vi "main.vi"() -> ()   [LabVIEW 2017]
uses:
  <vilib>/Instr/_visa.llb/VISA Configure Serial Port (Instr).vi
  <vilib>/Utility/file.llb/Write Delimited Spreadsheet (DBL).vi
  <vilib>/ptbypt/NI_PtbyPt.lvlib
panel:
  out "路径":path
  out "XY图":cluster{dbl[], dbl[]}(graph)
  out "激光位移传感器":dbl(graph)
  in  "模拟信号串口号":refnum<visa-resource-name>="COM12"
  out "读取缓冲区 2":string
  out "力传感器":cluster{dbl, dbl, dbl}(graph)
  out "Fz":dbl
  out "Fy":dbl
  out "Fx":dbl
  out "连接的字符串":string
  out "频率/Hz":dbl
  out "relative seconds":dbl caption="相对秒钟" format="%_19f"
  in  "六轴力传感器置零":bool
  in  "停止":bool
  in  "六轴力传感器串口号":refnum<visa-resource-name>="COM11"
  out "读取缓冲区":string
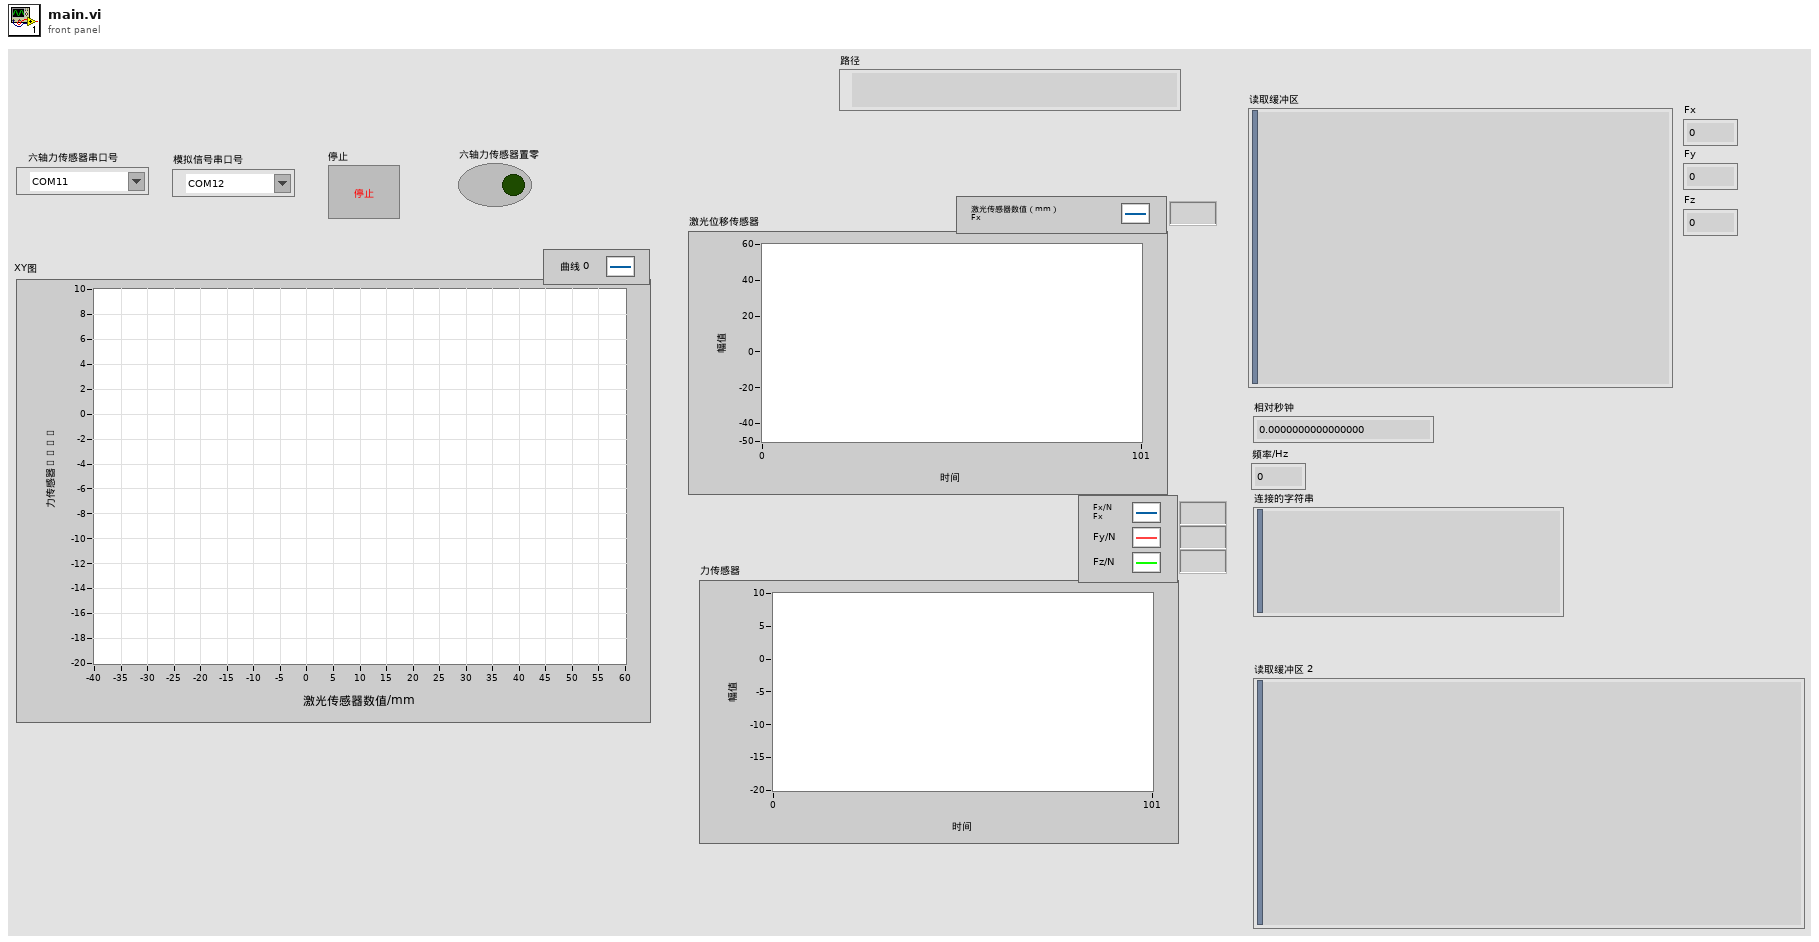
[diagram p1: front panel]
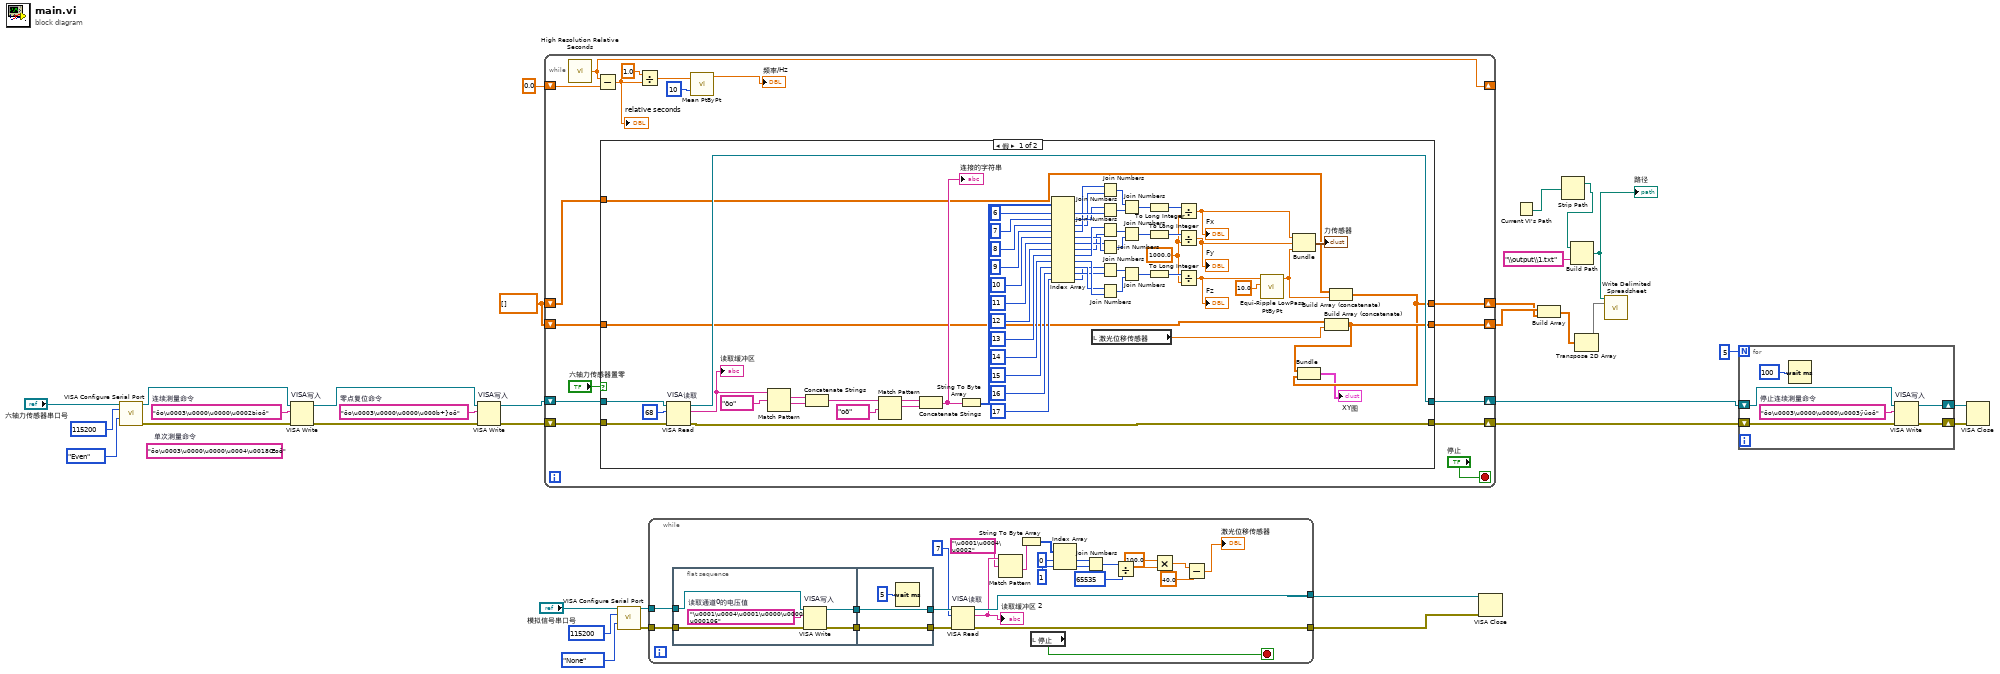
[diagram p0: block diagram]
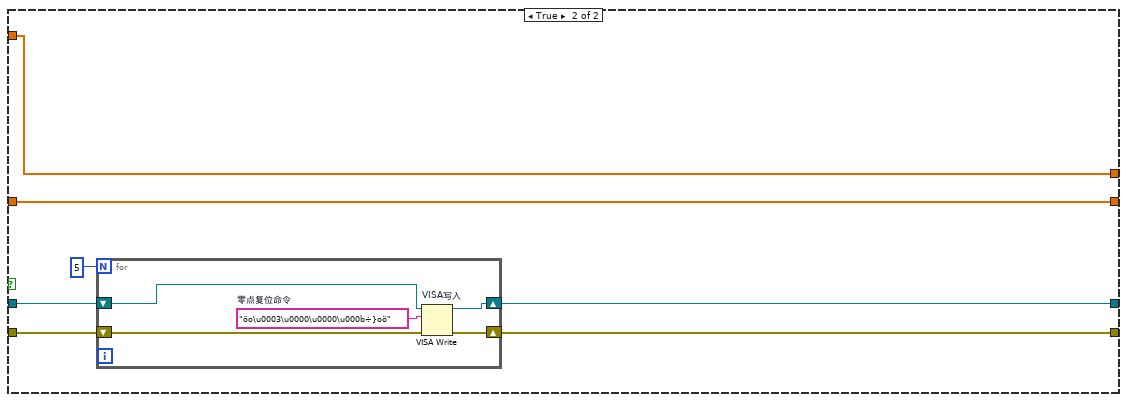
[diagram p2: hidden frame]
diagram:
  w9 = dbl[] []
  (unwired) "öo\u0003\u0000\u0000\u0004\u0018Œoö"  # 单次测量命令
  w23 = "öo\u0003\u0000\u0000\u000b÷}oö"  # 零点复位命令
  w17 = "öo\u0003\u0000\u0000\u0002Þìoö"  # 连续测量命令
  n1 = call-poly "VISA Configure Serial Port"("VISA resource name"="六轴力传感器串口号", "baud rate (9600)"=u32 115200, "parity (0:none)"=enum16{"None", "Odd", "Even", "Mark", "Space"}."Even") -> ("VISA resource name out"=w19:refnum<visa-resource-name>, "error out"=w21:errorcluster)  [unwired: 11 in]
  n2 = VISA Write "VISA写入"(VISA resource name=w19, write buffer=w17, error in (no error)=w21) -> (VISA resource name out=w18:refnum<visa-resource-name>, error out=w20:errorcluster)  [unwired: 1 out]
  n3 = VISA Write "VISA写入"(VISA resource name=w18, write buffer=w23, error in (no error)=w20) -> (VISA resource name out=w25:refnum<visa-resource-name>, error out=w24:errorcluster)  [unwired: 1 out]
  n4 = while {
    shift-right: [w50] -> w30
    shift-left: w25 -> [w39]
    shift-right: [w49] -> w29
    shift-left: w24 -> [w38]
    shift-right: [w46] -> _
    shift-left: 0.0 ("relative seconds") -> [w45]
    shift-right: [w37] -> w7
    shift-left: w9 -> [w36]
    shift-right: [w35] -> w8
    shift-left: w9 -> [w34]
    stop <- "停止" stop-if-true
    n5 = call <vilib>:"High Resolution Relative Seconds.vi"() -> ("relative seconds"=w46:dbl)
    n6 = Subtract(x=w46, y=w45) -> (x-y=w44:dbl)
    "relative seconds" <- w44
    n7 = case shown="假" "六轴力传感器置零" {
      tunnel: [w113 w120] -> w50
      tunnel: [w112 w121] -> w49
      tunnel: w39 -> [w59 w118]
      tunnel: w38 -> [w58 w117]
      tunnel: [w52 w116] -> w37
      tunnel: w36 -> [w56 w116]
      tunnel: [w53 w115] -> w35
      tunnel: w34 -> [w54 w115]
      frame False {
        w76 = 1000.0
        n8 = VISA Read "VISA读取"(VISA resource name=w59, byte count=u32 68 ("字节总数"), error in (no error)=w58) -> (VISA resource name out=w113:refnum<visa-resource-name>, read buffer=w111:string, error out=w112:errorcluster)  [unwired: 1 out]
        "读取缓冲区" <- w111
        n9 = Match Pattern(string=w111, regular expression="öo" ("正则表达式")) -> (match substring=w107:string, after substring=w106:string)  [unwired: 1 in, 2 out]
        n10 = Concatenate Strings(w107, w106) -> (w105:string)
        n11 = Match Pattern(string=w105, regular expression="oö" ("正则表达式")) -> (before substring=w103:string, match substring=w102:string)  [unwired: 1 in, 2 out]
        n12 = Concatenate Strings(w103, w102) -> (w101:string)
        "连接的字符串" <- w101
        n13 = String To Byte Array(string=w101) -> (unsigned byte array=w109:u8[])
        n14 = Index Array(array=w109, index #1=6 ("索引"), index #2=7 ("索引"), index #3=8 ("索引"), index #4=9 ("索引"), index #5=10 ("索引"), index #6=11 ("索引"), index #7=12 ("索引"), index #8=13 ("索引"), index #9=14 ("索引"), index #10=15 ("索引"), index #11=16 ("索引"), index #12=17 ("索引")) -> (element #1=w100:u8, element #2=w99:u8, element #3=w97:u8, element #4=w98:u8, element #5=w90:u8, element #6=w89:u8, element #7=w88:u8, element #8=w91:u8, element #9=w83:u8, element #10=w82:u8, element #11=w81:u8, element #12=w80:u8)
        n15 = local read "激光位移传感器"() -> (w55:dbl)
        n16 = Join Numbers(hi=w98, lo=w97) -> ((hi.lo)=w95:u16)
        n17 = Join Numbers(hi=w99, lo=w100) -> ((hi.lo)=w96:u16)
        n18 = Join Numbers(hi=w91, lo=w88) -> ((hi.lo)=w93:u16)
        n19 = Join Numbers(hi=w89, lo=w90) -> ((hi.lo)=w92:u16)
        n20 = Join Numbers(hi=w80, lo=w81) -> ((hi.lo)=w84:u16)
        n21 = Join Numbers(hi=w82, lo=w83) -> ((hi.lo)=w85:u16)
        n22 = Join Numbers(hi=w95, lo=w96) -> ((hi.lo)=w94:u32)
        n23 = Join Numbers(hi=w93, lo=w92) -> ((hi.lo)=w87:u32)
        n24 = Join Numbers(hi=w84, lo=w85) -> ((hi.lo)=w86:u32)
        n25 = To Long Integer(number=w94) -> (32bit integer=w79:i32)
        n26 = To Long Integer(number=w87) -> (32bit integer=w77:i32)
        n27 = To Long Integer(number=w86) -> (32bit integer=w78:i32)
        n28 = Divide(x=w79, y=w76) -> (x/y=w63:dbl)
        "Fx" <- w63
        n29 = Divide(x=w77, y=w76) -> (x/y=w62:dbl)
        "Fy" <- w62
        n30 = Divide(x=w78, y=w76) -> (x/y=w61:dbl)
        "Fz" <- w61
        n31 = call <vilib>:"Equi-Ripple LowPass PtByPt.vi"("sampling freq: fs"=10.0, "x"=w61) -> ("Filtered x"=w57:dbl)  [unwired: 7 in, 1 out]
        n32 = Bundle(w63, w62, "Filtered x"=w57) -> (→"力传感器":cluster{dbl, dbl, "Filtered x":dbl})  [unwired: 1 in]
        n33 = Build Array (concatenate)(w54, w55) -> (w53:dbl[])
        n34 = Build Array (concatenate)(w56, w57) -> (w52:dbl[])
        n35 = Bundle(w53, w52) -> (→"XY图":cluster{dbl[], dbl[]})  [unwired: 1 in]
      }
      frame True {
        n36 = for {
          N: 5 -> [_]
          shift-right: [w124] -> w121
          shift-left: w117 -> [w125]
          shift-right: [w122] -> w120
          shift-left: w118 -> [w123]
          w126 = "öo\u0003\u0000\u0000\u000b÷}oö"  # 零点复位命令
          n37 = VISA Write "VISA写入"(VISA resource name=w123, write buffer=w126, error in (no error)=w125) -> (VISA resource name out=w122:refnum<visa-resource-name>, error out=w124:errorcluster)  [unwired: 1 out]
        }
      }
    }
    n38 = Divide(x=1.0, y=w44) -> (x/y=w42:dbl)
    n39 = call <vilib>:"Mean PtByPt.vi"("x"=w42, "sample length"=10) -> ("mean"=→"频率/Hz":dbl)  [unwired: 2 in, 1 out]
  }
  n40 = call-poly "VISA Configure Serial Port"("VISA resource name"="模拟信号串口号", "baud rate (9600)"=u32 115200, "parity (0:none)"=enum16{"None", "Odd", "Even", "Mark", "Space"}."None") -> ("VISA resource name out"=w13:refnum<visa-resource-name>, "error out"=w12:errorcluster)  [unwired: 11 in]
  n41 = while {
    tunnel: w13 -> [w148]
    tunnel: w12 -> [w147]
    tunnel: [w146] -> w11
    tunnel: [w145] -> w10
    stop <- w142 stop-if-true
    n42 = flat-sequence {
      tunnel: w148 -> [w153]
      tunnel: w147 -> [w152]
      tunnel: [w156] -> w144
      tunnel: [w155] -> w143
      tunnel: w144 -> [w159]
      tunnel: w143 -> [w158]
      tunnel: [w159] -> w151
      tunnel: [w158] -> w150
      frame #0 {
        w154 = "\u0001\u0004\u0001\u0000\u0000\u000106"  # 读取通道0的电压值
        n43 = VISA Write "VISA写入"(VISA resource name=w153, write buffer=w154, error in (no error)=w152) -> (VISA resource name out=w155:refnum<visa-resource-name>, error out=w156:errorcluster)  [unwired: 1 out]
      }
      frame #1 {
        n44 = Wait (ms)(milliseconds to wait=u32 5 ("等待时间（毫秒）")) -> ()  [unwired: 1 out]
      }
    }
    n45 = VISA Read "VISA读取"(VISA resource name=w150, byte count=u32 7 ("字节总数"), error in (no error)=w151) -> (VISA resource name out=w146:refnum<visa-resource-name>, read buffer=w141:string, error out=w145:errorcluster)  [unwired: 1 out]
    "读取缓冲区 2" <- w141
    n46 = Match Pattern(string=w141, regular expression="\u0001\u0004\u0002" ("正则表达式")) -> (after substring=w137:string)  [unwired: 1 in, 3 out]
    n47 = String To Byte Array(string=w137) -> (unsigned byte array=w136:u8[])
    n48 = local read "停止"() -> (w142:bool)
    n49 = Index Array(array=w136, index #1=0 ("索引"), index #2=1 ("索引")) -> (element #1=w134:u8, element #2=w135:u8)
    n50 = Join Numbers(hi=w134, lo=w135) -> ((hi.lo)=w133:u16)
    n51 = Divide(x=w133, y=u16 65535) -> (x/y=w131:dbl)
    n52 = Multiply(x=100.0, y=w131) -> (x*y=w129:dbl)
    n53 = Subtract(x=w129, y=40.0) -> (x-y=→"激光位移传感器":dbl)
  }
  n54 = VISA Close(VISA resource name=w11, error in (no error)=w10) -> ()  [unwired: 1 out]
  n55 = Current VI's Path() -> (path=w3:path)
  n56 = Build Array(w8, w7) -> (w6:dbl[][])
  n57 = Strip Path(path=w3) -> (stripped path=w2:path)  [unwired: 1 out]
  n58 = Build Path(base path=w2, name or relative path="\\output\\1.txt" ("名称或相对路径")) -> (appended path=w1:path)
  "路径" <- w1
  n59 = Transpose 2D Array(2D array=w6) -> (transposed array=w5:dbl[][])
  n60 = call-poly <vilib>:"Write Delimited Spreadsheet.vi"("file path (dialog if empty)"=w1, "2D data"=w5) -> ()  [unwired: 12 in, 2 out]
  n61 = for {
    N: 5 -> [_]
    shift-right: [w162] -> w27
    shift-left: w30 -> [w165]
    shift-right: [w163] -> w28
    shift-left: w29 -> [w164]
    w161 = "öo\u0003\u0000\u0000\u0003ÿüoö"  # 停止连续测量命令
    n62 = Wait (ms)(milliseconds to wait=u32 100 ("等待时间（毫秒）")) -> ()  [unwired: 1 out]
    n63 = VISA Write "VISA写入"(VISA resource name=w165, write buffer=w161, error in (no error)=w164) -> (VISA resource name out=w162:refnum<visa-resource-name>, error out=w163:errorcluster)  [unwired: 1 out]
  }
  n64 = VISA Close(VISA resource name=w27, error in (no error)=w28) -> ()  [unwired: 1 out]
